vi "lorentzian transformations--test.vi"() -> ()   [LabVIEW 2020]
uses:
  lorentzian.ctl
  circle corners.ctl
  cursor action.ctl
  four-corner circle transformation.ctl
  Q -- check range -- i -- real.vi
  draw a line.vi
  draw a circle.vi
  Q - not nan -- real.vi
  generate linear region.vi
panel:
  in  "lorentzian hist":T1={"A (VHz)"=1.0, "f (Hz)"=900.0, "G (Hz)"=10.0, "phi(rad)"=0.0, "Q"=0.006429595340103388, "Norm  Ampl"=nan, "bg (V)"=0.0+0.0i, "4corners"={"z (-pi/2)"=0.1-0.1i, "z(inf)"=0.0+0.0i, "z (pi/2)"=-0.1-0.1i, "z center"=0.0-0.1i, "z(0)"=0.0-0.2i, "radius"=0.1}} {"bg (V)" format="%#9_9f"; "Q" format="%#9_9f"; "phi(rad)" format="%#9_9f"; "G (Hz)" format="%#9_9f"; "f (Hz)" format="%#9_9f"}
  in  "Tab Control":enum32{"Page 1", "Page 2"}(tab)
  in  "phase":dbl(slide) scale=-1.57..1.57
  out "Plot: complex plane":cluster{dbl[], dbl[]}[](graph)=[{[0.1, 0.09991228300988585, 0.09964928592495044, 0.0992114701314478, 0.0985996037070505, 0.09781476007338057, 0.09685831611286312, 0.09573194975320673, 0.0944376370237481, 0.09297764858882515, 0.0913545457642601, 0.0895711760239413, 0.08763066800438636, 0.08553642601605067, 0.08329212407100996, 0.08090169943749474, 0.07836934573258399, 0.07569950556517566, 0.07289686274214116, 0.06996633405133655, 0.06691306063588583, 0.06374239897486898, 0.06045991148623749, 0.05707135676844318, 0.05358267949789968, 0.05000000000000001, 0.04632960351198618, 0.04257792915650729, 0.038751558645210314, 0.03485720473218153, 0.03090169943749475, 0.02689198206152659, 0.02283508701106559, 0.018738131458572473, 0.014608302856241187, 0.010452846326765368, 0.006279051952931353, 0.002094241988335705, -0.0020942419883356704, -0.006279051952931318, -0.010452846326765334, -0.014608302856241132, -0.01873813145857244, -0.02283508701106556, -0.02689198206152656, -0.030901699437494715, -0.0348572047321815, -0.03875155864521028, -0.04257792915650724, -0.04632960351198615, -0.04999999999999998, -0.05358267949789965, -0.05707135676844316, -0.060459911486237486, -0.06374239897486894, -0.0669130606358858, -0.06996633405133652, -0.07289686274214113, -0.07569950556517563, -0.07836934573258397, -0.08090169943749474, -0.08329212407100993, -0.08553642601605065, -0.08763066800438635, -0.08957117602394128, -0.09135454576426008, -0.09297764858882514, -0.0944376370237481, -0.09573194975320672, -0.09685831611286311, -0.09781476007338057, -0.0985996037070505, -0.09921147013144778, -0.09964928592495044, -0.09991228300988585, -0.1, -0.09991228300988585, -0.09964928592495044, -0.0992114701314478, -0.09859960370705051, -0.09781476007338058, -0.09685831611286312, -0.09573194975320674, -0.09443763702374813, -0.09297764858882517, -0.09135454576426011, -0.08957117602394131, -0.08763066800438638, -0.08553642601605069, -0.08329212407100998, -0.08090169943749478, -0.07836934573258401, -0.07569950556517568, -0.07289686274214119, -0.06996633405133657, -0.06691306063588585, -0.06374239897486902, -0.06045991148623754, -0.05707135676844322, -0.05358267949789971, -0.050000000000000044, -0.046329603511986214, -0.0425779291565073, -0.03875155864521033, -0.03485720473218155, -0.03090169943749476, -0.026891982061526584, -0.022835087011065666, -0.01873813145857255, -0.014608302856241245, -0.010452846326765424, -0.006279051952931409, -0.002094241988335762, 0.002094241988335636, 0.006279051952931284, 0.010452846326765299, 0.01460830285624112, 0.018738131458572428, 0.022835087011065545, 0.026891982061526546, 0.030901699437494726, 0.03485720473218143, 0.03875155864521021, 0.04257792915650718, 0.0463296035119861, 0.04999999999999993, 0.053582679497899605, 0.05707135676844312, 0.06045991148623744, 0.06374239897486893, 0.06691306063588578, 0.06996633405133651, 0.07289686274214113, 0.07569950556517563, 0.07836934573258397, 0.08090169943749473, 0.0832921240710099, 0.08553642601605062, 0.08763066800438632, 0.08957117602394125, 0.09135454576426007, 0.09297764858882512, 0.09443763702374809, 0.09573194975320672, 0.09685831611286311, 0.09781476007338055, 0.0985996037070505, 0.09921147013144778, 0.09964928592495044, 0.09991228300988583], [-0.1, -0.09581243462708004, -0.09163221566676846, -0.08746667664356958, -0.08332312532838979, -0.07920883091822407, -0.07513101128351453, -0.07109682030555285, -0.0671133353261417, -0.06318754473153221, -0.05932633569241998, -0.05553648208150726, -0.05182463258982848, -0.04819729906268699, -0.0446608450756656, -0.04122147477075269, -0.037885221972168974, -0.034657939600989465, -0.03154528940713114, -0.02855273203671968, -0.02568551745226058, -0.022948675722421083, -0.020347008197580382, -0.017885079086629604, -0.015567207449798504, -0.01339745962155614, -0.011379642076878527, -0.009517294753398062, -0.007813684841149957, -0.006271801050810849, -0.00489434837048465, -0.0036837433202341896, -0.002642109712683971, -0.001771274927131139, -0.0010727667037011696, -0.0005478104631726627, -0.00019732715717284133, -2.1931652515447264e-05, -2.1931652515447264e-05, -0.00019732715717284133, -0.0005478104631726627, -0.0010727667037011696, -0.0017712749271311251, -0.002642109712683971, -0.0036837433202341757, -0.004894348370484636, -0.006271801050810835, -0.007813684841149943, -0.009517294753398034, -0.011379642076878513, -0.013397459621556126, -0.01556720744979849, -0.01788507908662959, -0.02034700819758037, -0.022948675722421055, -0.025685517452260553, -0.02855273203671964, -0.03154528940713111, -0.03465793960098944, -0.03788522197216895, -0.041221474770752685, -0.044660845075665555, -0.048197299062686945, -0.051824632589828445, -0.05553648208150723, -0.05932633569241996, -0.06318754473153218, -0.06711333532614167, -0.0710968203055528, -0.07513101128351449, -0.07920883091822403, -0.08332312532838974, -0.08746667664356955, -0.09163221566676844, -0.09581243462708003, -0.09999999999999995, -0.10418756537291991, -0.1083677843332315, -0.11253332335643039, -0.1166768746716102, -0.12079116908177591, -0.12486898871648547, -0.12890317969444712, -0.1328866646738583, -0.13681245526846775, -0.14067366430758, -0.1444635179184927, -0.1481753674101715, -0.15180270093731302, -0.15533915492433437, -0.15877852522924726, -0.162114778027831, -0.1653420603990105, -0.16845471059286884, -0.1714472679632803, -0.1743144825477394, -0.1770513242775789, -0.17965299180241961, -0.1821149209133704, -0.1844327925502015, -0.18660254037844387, -0.18862035792312146, -0.19048270524660194, -0.19218631515885004, -0.19372819894918913, -0.19510565162951538, -0.19631625667976582, -0.197357890287316, -0.19822872507286887, -0.19892723329629883, -0.19945218953682733, -0.19980267284282716, -0.19997806834748455, -0.19997806834748455, -0.19980267284282716, -0.19945218953682736, -0.19892723329629886, -0.19822872507286887, -0.19735789028731604, -0.19631625667976582, -0.19510565162951538, -0.1937281989491892, -0.1921863151588501, -0.190482705246602, -0.18862035792312154, -0.18660254037844393, -0.18443279255020156, -0.18211492091337045, -0.17965299180241967, -0.17705132427757897, -0.17431448254773946, -0.17144726796328036, -0.1684547105928689, -0.16534206039901056, -0.16211477802783106, -0.15877852522924735, -0.1553391549243345, -0.15180270093731313, -0.14817536741017162, -0.14446351791849282, -0.1406736643075801, -0.13681245526846786, -0.1328866646738584, -0.12890317969444723, -0.12486898871648554, -0.12079116908177599, -0.11667687467161028, -0.11253332335643047, -0.10836778433323159, -0.10418756537292]}, {[0.0, 0.0, 0.0, 0.0, 0.0, 0.0, 0.0, 0.0, 0.0, 0.0, 0.0, 0.0, 0.0, 0.0, 0.0, 0.0, 0.0, 0.0, 0.0, 0.0], [0.0, -0.01, -0.02, -0.03, -0.04, -0.05, -0.06, -0.07, -0.08, -0.09, -0.1, -0.11, -0.12, -0.13, -0.14, -0.15, -0.16, -0.17, -0.18, -0.19]}, {[0.1, 0.09000000000000001, 0.08, 0.07, 0.060000000000000005, 0.05, 0.04000000000000001, 0.03, 0.020000000000000004, 0.010000000000000009, 0.0, -0.009999999999999995, -0.01999999999999999, -0.03, -0.04000000000000001, -0.04999999999999999, -0.06, -0.07, -0.07999999999999999, -0.09], [-0.1, -0.1, -0.1, -0.1, -0.1, -0.1, -0.1, -0.1, -0.1, -0.1, -0.1, -0.1, -0.1, -0.1, -0.1, -0.1, -0.1, -0.1, -0.1, -0.1]}, {[0.2, 0.18000000000000002, 0.16, 0.14, 0.12000000000000001, 0.1, 0.08000000000000002, 0.06, 0.04000000000000001, 0.020000000000000018, 0.0, -0.01999999999999999, -0.03999999999999998, -0.06, -0.08000000000000002, -0.09999999999999998, -0.12, -0.14, -0.15999999999999998, -0.18], [-1.2246063538223773e-17, -1.2246063538223773e-17, -1.2246063538223773e-17, -1.2246063538223773e-17, -1.2246063538223773e-17, -1.2246063538223773e-17, -1.2246063538223773e-17, -1.2246063538223773e-17, -1.2246063538223773e-17, -1.2246063538223773e-17, -1.2246063538223773e-17, -1.2246063538223773e-17, -1.2246063538223773e-17, -1.2246063538223773e-17, -1.2246063538223773e-17, -1.2246063538223773e-17, -1.2246063538223773e-17, -1.2246063538223773e-17, -1.2246063538223773e-17, -1.2246063538223773e-17]}]
  in  "lorentzian":T1={"A (VHz)"=1.0, "f (Hz)"=900.0, "G (Hz)"=10.0, "phi(rad)"=0.0, "Q"=0.006429595340103388, "Norm  Ampl"=nan, "bg (V)"=0.0+0.0i, "4corners"={"z (-pi/2)"=0.1-0.1i, "z(inf)"=0.0+0.0i, "z (pi/2)"=-0.1-0.1i, "z center"=0.0-0.1i, "z(0)"=0.0-0.2i, "radius"=0.1}} {"bg (V)" format="%#9_9f"; "Q" format="%#9_9f"; "phi(rad)" format="%#9_9f"; "G (Hz)" format="%#9_9f"; "f (Hz)" format="%#9_9f"}
  in  "exit":bool
  in  "omega":dbl(slide)=911.4832535885167 scale=500.0..1500.0
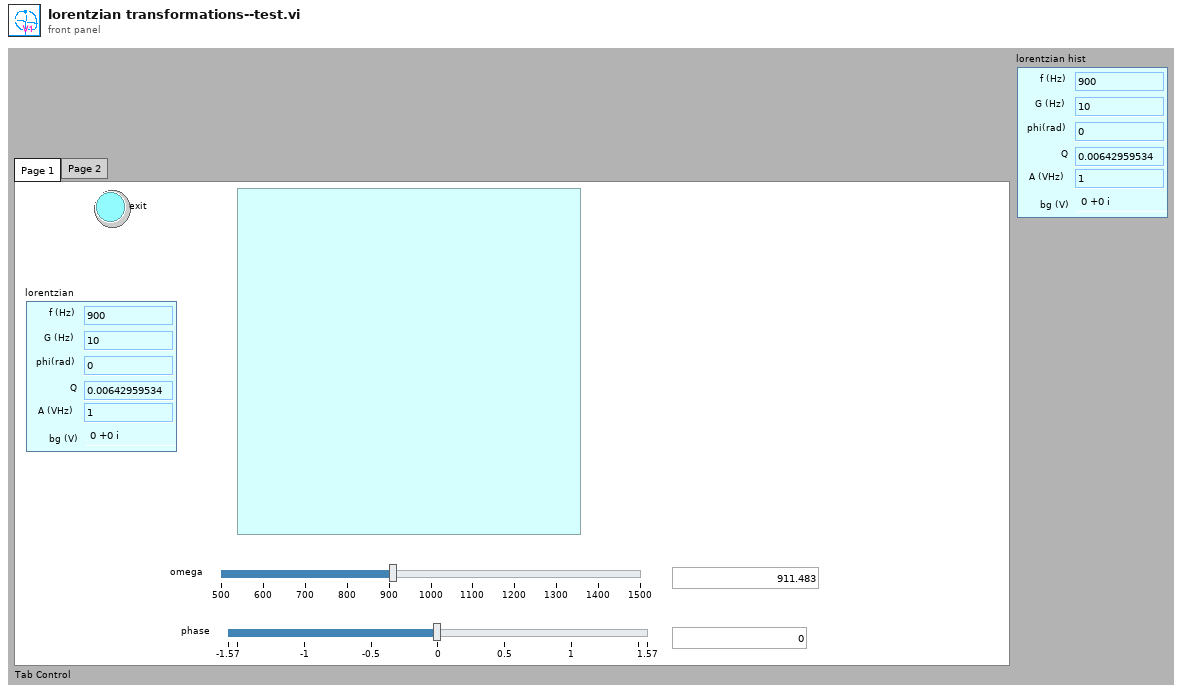
[diagram p1: front panel]
types:
  T1 = typedef "lorentzian.ctl" = cluster{"A (VHz)":dbl, "f (Hz)":dbl, "G (Hz)":dbl, "phi(rad)":dbl, "Q":dbl, "Norm  Ampl":dbl, "bg (V)":cdb, "4corners":T2}
  T2 = typedef "circle corners.ctl" = cluster{"z (-pi/2)":cdb, "z(inf)":cdb, "z (pi/2)":cdb, "z center":cdb, "z(0)":cdb, "radius":dbl}
  T3 = typedef "four-corner circle transformation.ctl" = enum16{"z(c) z(inf)", "z(c) z(zero)", "fix phase", "calculate lorentzian", "z(0) z(+-pi/2)", "shift to zcenter", "to  canonical", "get canonical phase", "get4corners", "update lorentzian -- from z0", "fake gamma normal", "fake gamma heat", "calculate complex slope", "get f0 given f and phi"}
  T4 = typedef "cursor action.ctl" = enum16{"range", "read", "write", "check", "zoom out", "smart zoom out", "zoom to aspect ratio 1", "zoom to win", "zoom out 20%", "zoom in 20%", "-empty", "smart zoom out&aspect", "move range left 20%", "move range right 20%", "move range up 20%", "move range down 20%", "zoom to X win", "zoom to Y win", "zoom out X", "zoom out Y", "zoom in X", "zoom in Y", "check plot scale"}
  T5 = typedef "eventvkey.ctl" = enum16{"ASCII", "Enter", "Return", "Shift", "Ctrl", "Alt", "Cmd", "Opt", "Caps", "NumLock", "Clear", "Break", "Up", "Down", "Left", "Right", "Insert", "Delete", "Home", "End", "PageUp", "PageDown", "Escape", "Help", "Pause", "ScrollLock", "F1", "F2", "F3", "F4", "F5", "F6", "F7", "F8", "F9", "F10", "F11", "F12", "F13", "F14", "F15", "F16", "F17", "F18", "F19", "F20", "F21", "F22", "F23", "F24", "Play", "VolumeUp", "VolumeDown", "Mute", "Two Byte Char"}
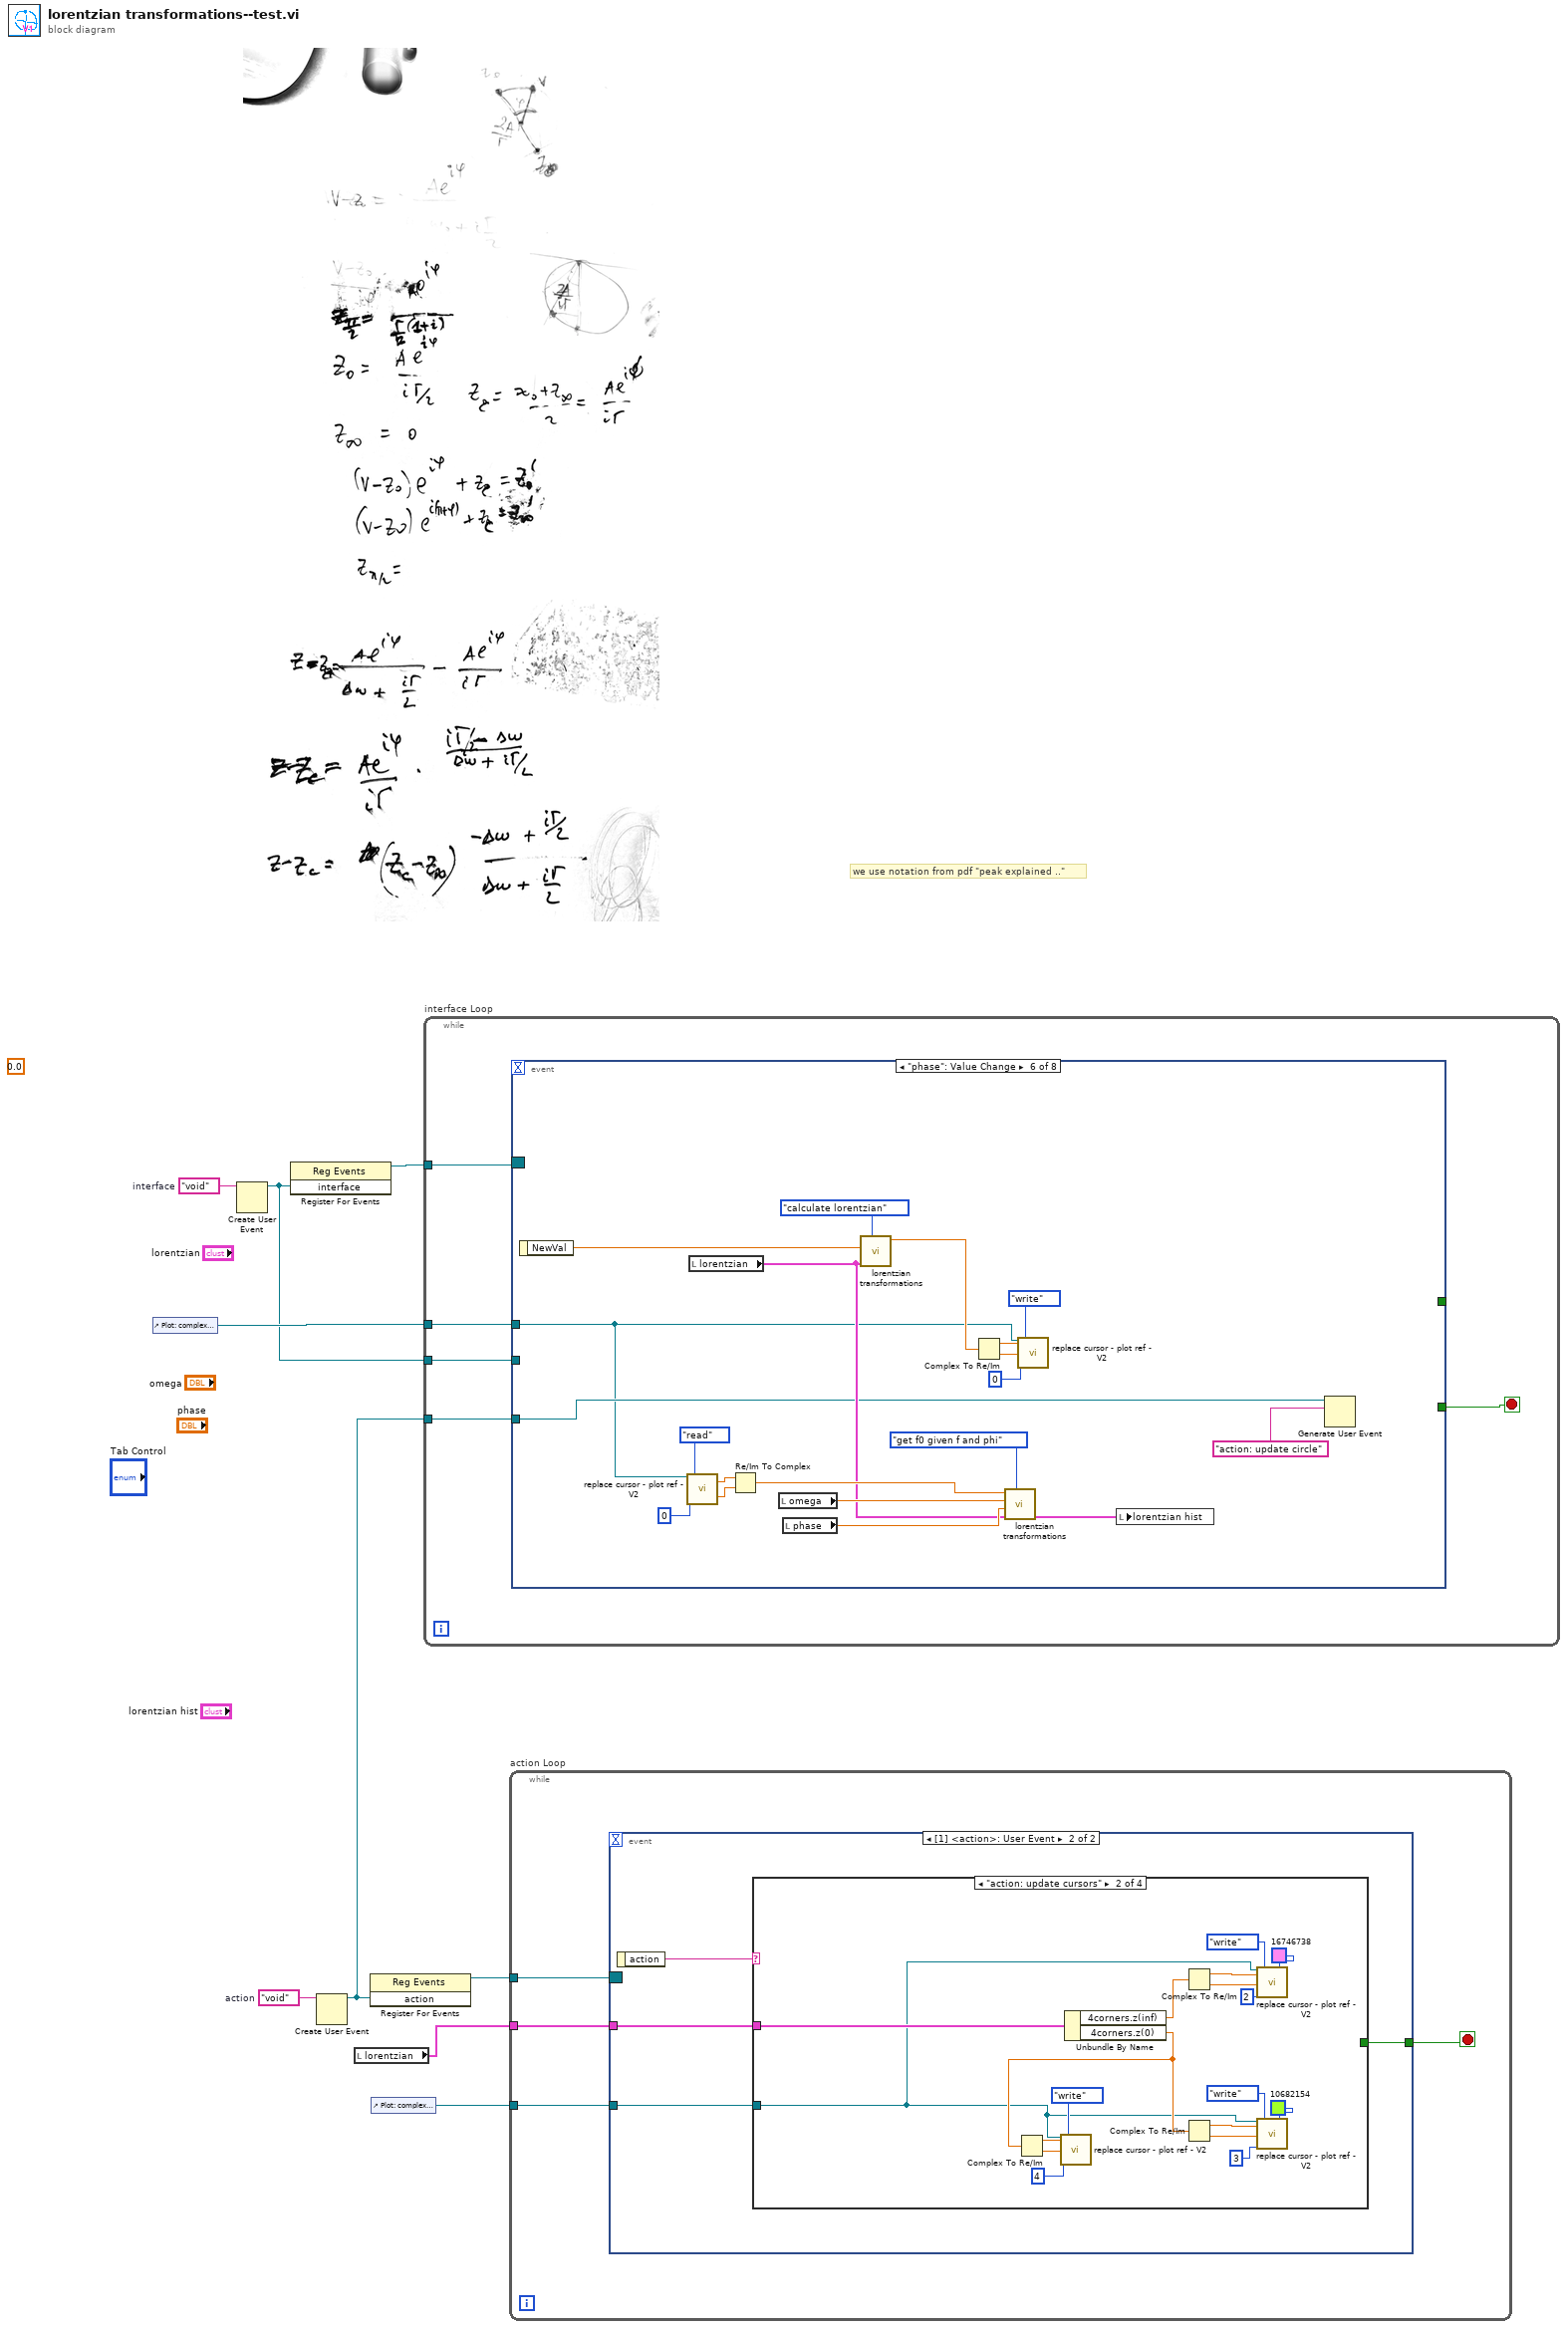
[diagram p0: block diagram]
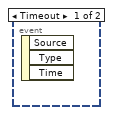
[diagram p2: hidden frame]
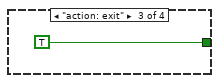
[diagram p4: hidden frame]
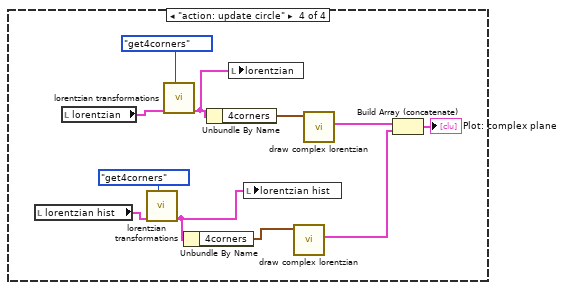
[diagram p5: hidden frame]
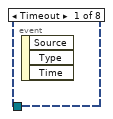
[diagram p6: hidden frame]
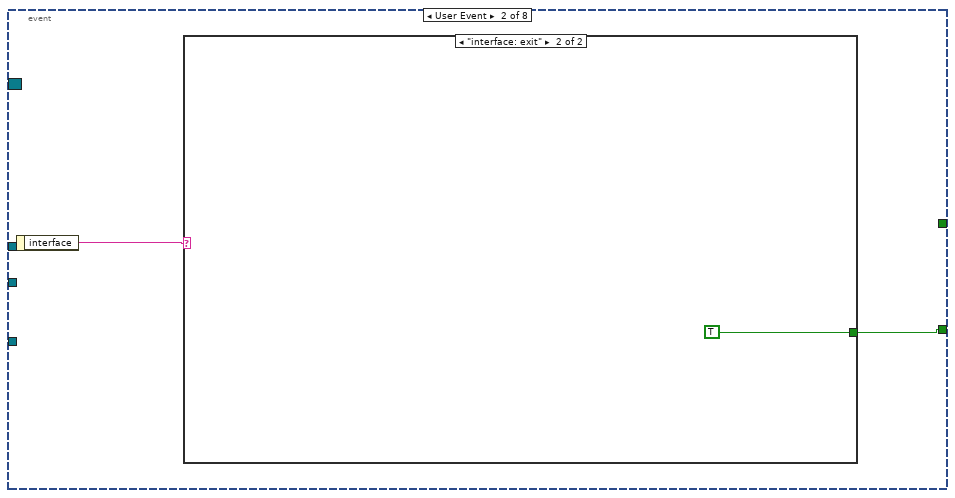
[diagram p7: hidden frame]
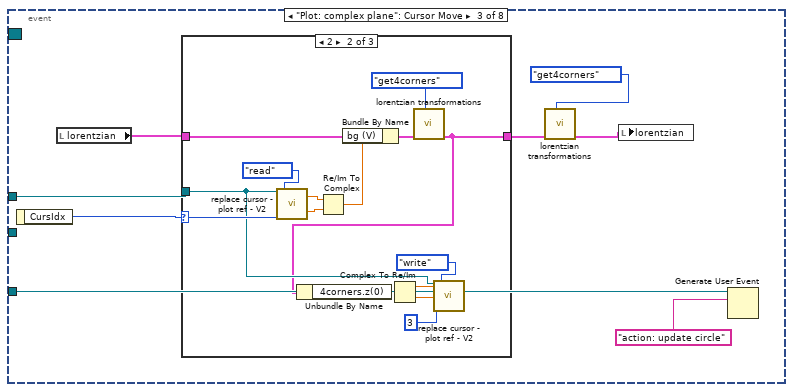
[diagram p9: hidden frame]
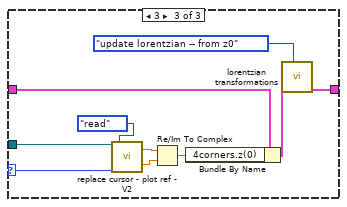
[diagram p11: hidden frame]
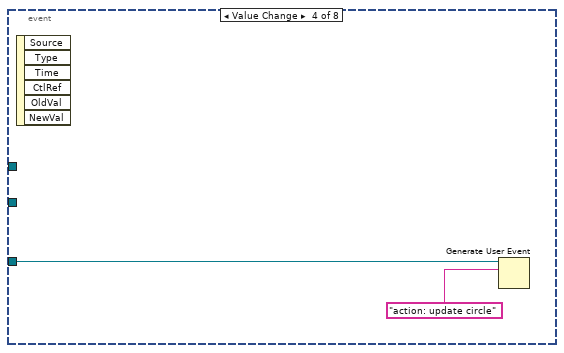
[diagram p12: hidden frame]
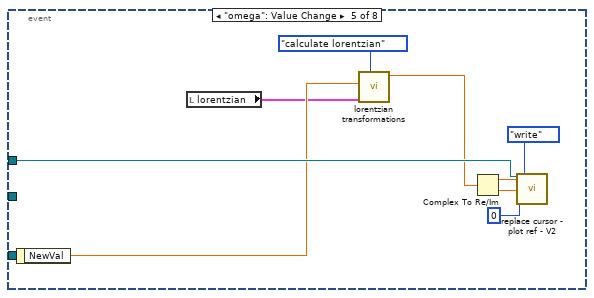
[diagram p13: hidden frame]
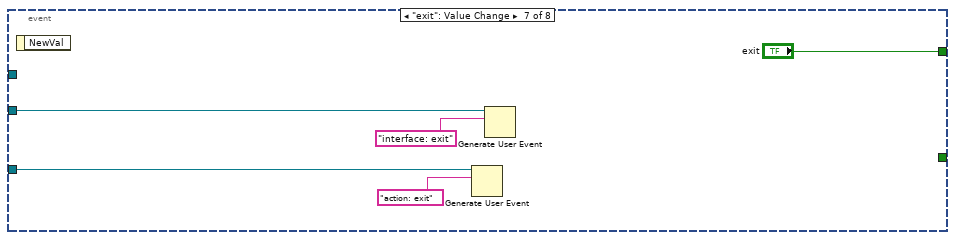
[diagram p14: hidden frame]
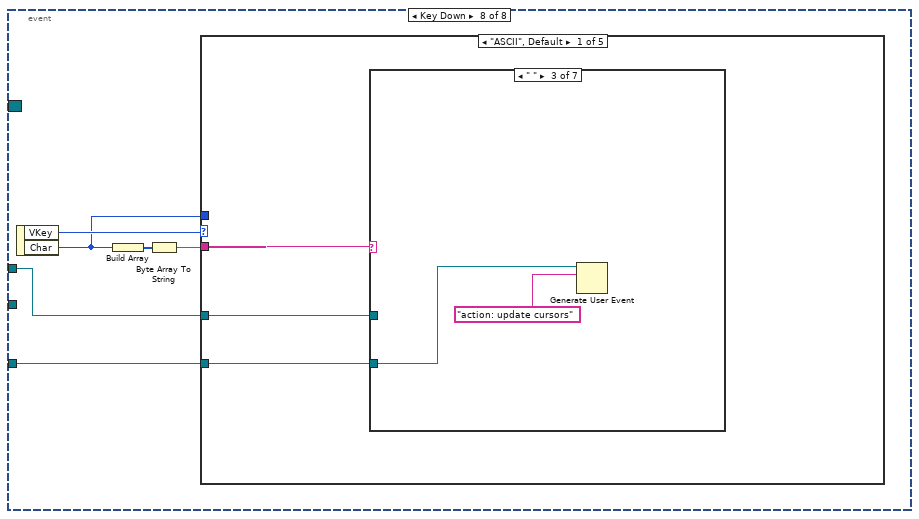
[diagram p15: hidden frame]
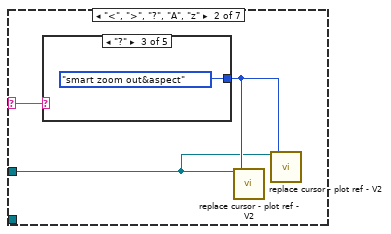
[diagram p17: hidden frame]
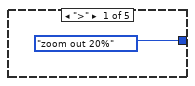
[diagram p18: hidden frame]
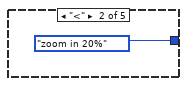
[diagram p19: hidden frame]
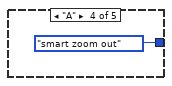
[diagram p20: hidden frame]
diagram:
  w5 = "void"  # interface
  w9 = "void"  # action
  (unwired) 0.0 ("zi phase temporary")
  # "we use notation from pdf \"peak explained ..\""
  n1 = control-ref of="Plot: complex plane"() -> (w2:refnum<vi>)
  n2 = Create User Event(user event datatype=w5) -> (user event=w1:refnum<user-event>)  [unwired: 1 in, 1 out]
  n3 = register-events(w1) -> (reference out=w4:refnum<event-registration>)  [unwired: 2 in, 1 out]
  n4 = Create User Event(user event datatype=w9) -> (user event=w3:refnum<user-event>)  [unwired: 1 in, 1 out]
  n5 = local read "lorentzian"() -> (w6:T1)
  n6 = register-events(w3) -> (reference out=w8:refnum<event-registration>)  [unwired: 2 in, 1 out]
  n7 = control-ref of="Plot: complex plane"() -> (w7:refnum<vi>)
  n8 = while "interface Loop" {
    tunnel: w4 -> [w14]
    tunnel: w3 -> [w13]
    tunnel: w2 -> [w12]
    tunnel: w1 -> [w10]
    stop <- w11 stop-if-true
    n9 = event shown="[5] \"phase\": Value Change" {
      selector: w14 -> [_ _ _ _ _ _ _ _]
      dyn-events: _ -> [_ _ _ _ _ _ _ _]
      timeout: _ -> [_ _ _ _ _ _ _ _]
      tunnel: [_ _ _ _ _ _ "exit" _] -> _
      tunnel: w13 -> [_ _ w18 w52 _ w64 w85 w88]
      tunnel: w12 -> [_ _ w22 _ w57 w63 _ w89]
      tunnel: [_ w15 _ _ _ _ _ _] -> w11
      tunnel: w10 -> [_ _ _ _ _ _ w83 _]
      event Timeout {
        n10 = event-data() -> ()  [unwired: 1 in, 3 out]
      }
      event User Event {
        n11 = event-data() -> ("interface"=w16:string)  [unwired: 1 in]
        n12 = case shown="\"interface: exit\"" w16 {
          tunnel: [_ TRUE] -> w15
          frame "False", Default {
          }
          frame "interface: exit" {
          }
        }
      }
      event "Plot: complex plane": Cursor Move {
        n13 = event-data() -> ("CursIdx"=w21:i32)  [unwired: 1 in]
        n14 = local read "lorentzian"() -> (w23:T1)
        n15 = case shown="2" w21 {
          selector: w21 -> [_ w37 w47]
          tunnel: w22 -> [_ w31 w46]
          tunnel: w23 -> [w26 w27 w45]
          tunnel: [w26 w28 w42] -> w25
          frame 0, Default {
          }
          frame 2 {
            n16 = call "replace cursor - plot ref - V2.vi"("Plot ref in"=w31, "cursor index"=w37, "cursor action"=cursor_action."read") -> ("read X"=w39:dbl, "read Y"=w40:dbl)  [unwired: 13 in, 2 out]
            n17 = Re/Im To Complex(1:w40, 2:w39) -> (0:w38:cdb)
            n18 = Bundle By Name(cluster=w27, "bg (V)"=w38) -> (w36:T1)
            n19 = call "lorentzian transformations.vi"("4 corner circle transformation"=four-corner_circle_transformation."get4corners", "lorentzian in"=w36) -> ("lorentzian out"=w28:T1)  [unwired: 6 in, 3 out]
            n20 = Unbundle By Name(w28) -> ("4corners.z(0)"=w34:cdb)
            n21 = Complex To Re/Im(x + iy=w34) -> (x=w33:dbl, y=w32:dbl)
            n22 = call "replace cursor - plot ref - V2.vi"("Plot ref in"=w31, "new X"=w33, "new  Y"=w32, "cursor index"=3, "cursor action"=cursor_action."write") -> ()  [unwired: 11 in, 4 out]
          }
          frame 3 {
            n23 = call "replace cursor - plot ref - V2.vi"("Plot ref in"=w46, "cursor index"=w47, "cursor action"=cursor_action."read") -> ("read X"=w49:dbl, "read Y"=w50:dbl)  [unwired: 13 in, 2 out]
            n24 = Re/Im To Complex(1:w50, 2:w49) -> (0:w48:cdb)
            n25 = Bundle By Name(cluster=w45, "4corners.z(0)"=w48) -> (w44:T1)
            n26 = call "lorentzian transformations.vi"("4 corner circle transformation"=four-corner_circle_transformation."update lorentzian -- from z0", "lorentzian in"=w44) -> ("lorentzian out"=w42:T1)  [unwired: 6 in, 3 out]
          }
        }
        n27 = call "lorentzian transformations.vi"("4 corner circle transformation"=four-corner_circle_transformation."get4corners", "lorentzian in"=w25) -> ("lorentzian out"=w20:T1)  [unwired: 6 in, 3 out]
        n28 = local write "lorentzian"(w20) -> ()
        n29 = Generate User Event(user event=w18, event data cluster="action: update circle" ("event data")) -> ()  [unwired: 2 in, 2 out]
      }
      event Value Change {
        n30 = event-data() -> ()  [unwired: 1 in, 6 out]
        n31 = Generate User Event(user event=w52, event data cluster="action: update circle" ("event data")) -> ()  [unwired: 2 in, 2 out]
      }
      event "omega": Value Change {
        n32 = event-data() -> ("NewVal"=w55:dbl)  [unwired: 1 in]
        n33 = local read "lorentzian"() -> (w54:T1)
        n34 = call "lorentzian transformations.vi"("4 corner circle transformation"=four-corner_circle_transformation."calculate lorentzian", "lorentzian in"=w54, "freq in"=w55) -> ("voltage out"=w56:cdb)  [unwired: 5 in, 3 out]
        n35 = Complex To Re/Im(x + iy=w56) -> (x=w61:dbl, y=w60:dbl)
        n36 = call "replace cursor - plot ref - V2.vi"("Plot ref in"=w57, "new X"=w61, "new  Y"=w60, "cursor index"=0, "cursor action"=cursor_action."write") -> ()  [unwired: 11 in, 4 out]
      }
      event "phase": Value Change {
        n37 = event-data() -> ("NewVal"=w76:dbl)  [unwired: 1 in]
        n38 = call "replace cursor - plot ref - V2.vi"("Plot ref in"=w63, "cursor index"=0, "cursor action"=cursor_action."read") -> ("read X"=w71:dbl, "read Y"=w72:dbl)  [unwired: 13 in, 2 out]
        n39 = local read "lorentzian"() -> (w68:T1)
        n40 = Re/Im To Complex(1:w72, 2:w71) -> (0:w70:cdb)
        n41 = local read "omega"() -> (w75:dbl)
        n42 = local read "phase"() -> (w69:dbl)
        n43 = call "lorentzian transformations.vi"("4 corner circle transformation"=four-corner_circle_transformation."calculate lorentzian", "lorentzian in"=w68, "freq in"=w76) -> ("voltage out"=w77:cdb)  [unwired: 5 in, 3 out]
        n44 = Complex To Re/Im(x + iy=w77) -> (x=w81:dbl, y=w80:dbl)
        n45 = call "lorentzian transformations.vi"("4 corner circle transformation"=four-corner_circle_transformation."get f0 given f and phi", "lorentzian in"=w68, "phase in (rad)"=w69, "freq in"=w75, "voltage in"=w70) -> ("lorentzian out"=w67:T1)  [unwired: 3 in, 3 out]
        n46 = call "replace cursor - plot ref - V2.vi"("Plot ref in"=w63, "new X"=w81, "new  Y"=w80, "cursor index"=0, "cursor action"=cursor_action."write") -> ()  [unwired: 11 in, 4 out]
        n47 = local write "lorentzian hist"(w67) -> ()
        n48 = Generate User Event(user event=w64, event data cluster="action: update circle" ("event data")) -> ()  [unwired: 2 in, 2 out]
      }
      event "exit": Value Change {
        n49 = event-data() -> ()  [unwired: 1 in, 1 out]
        n50 = Generate User Event(user event=w85, event data cluster="action: exit" ("event data")) -> ()  [unwired: 2 in, 2 out]
        n51 = Generate User Event(user event=w83, event data cluster="interface: exit" ("event data")) -> ()  [unwired: 2 in, 2 out]
      }
      event Key Down {
        n52 = event-data() -> ("VKey"=w91:T5, "Char"=w90:i16)  [unwired: 1 in]
        n53 = Build Array(w90) -> (w93:i16[])
        n54 = Byte Array To String(unsigned byte array=w93) -> (string=w92:string)
        n55 = case shown="\"ASCII\", Default" w91 {
          selector: w91 -> [_ _ _ _ w109]
          tunnel: w90 -> [_ _ _ _ _]
          tunnel: w92 -> [w96 _ _ _ _]
          tunnel: w89 -> [w95 _ _ _ w107]
          tunnel: w88 -> [w94 _ _ _ _]
          frame "ASCII", Default {
            n56 = case shown="\" \"" w96 {
              selector: w96 -> [_ w98 _ _ _ _ _]
              tunnel: w95 -> [_ w97 _ _ _ _ _]
              tunnel: w94 -> [_ _ w105 _ _ _ _]
              frame "0", Default {
              }
              frame "<", ">", "?", "A", "z" {
                n57 = case shown="\"?\"" w98 {
                  tunnel: [cursor_action."zoom out 20%" ("cursor action") cursor_action."zoom in 20%" ("cursor action") cursor_action."smart zoom out&aspect" ("cursor action") cursor_action."smart zoom out" ("cursor action") cursor_action."zoom to aspect ratio 1" ("cursor action")] -> w99
                  frame ">" {
                  }
                  frame "<" {
                  }
                  frame "?" {
                  }
                  frame "A" {
                  }
                  frame "z", Default {
                  }
                }
                n58 = call "replace cursor - plot ref - V2.vi"("Plot ref in"=w97, "cursor action"=w99) -> ()  [unwired: 14 in, 4 out]
                n59 = call "replace cursor - plot ref - V2.vi"("Plot ref in"=w97, "cursor action"=w99) -> ()  [unwired: 14 in, 4 out]
              }
              frame " " {
                n60 = Generate User Event(user event=w105, event data cluster="action: update cursors" ("event data")) -> ()  [unwired: 2 in, 2 out]
              }
              frame "'", ";", "[", "]", "{", "}" {
              }
              frame "@" {
              }
              frame "#" {
              }
              frame "q" {
              }
            }
          }
          frame "Escape" {
          }
          frame "PageUp" {
          }
          frame "PageDown" {
          }
          frame "Up".."Right" {
            n61 = case shown="\"Down\"" w109 {
              tunnel: [cursor_action."move range right 20%" ("cursor action") cursor_action."move range left 20%" ("cursor action") cursor_action."move range up 20%" ("cursor action") cursor_action."move range down 20%" ("cursor action")] -> w108
              frame "Right", Default {
              }
              frame "Left" {
              }
              frame "Up" {
              }
              frame "Down" {
              }
            }
            n62 = call "replace cursor - plot ref - V2.vi"("Plot ref in"=w107, "cursor action"=w108) -> ()  [unwired: 14 in, 4 out]
            n63 = call "replace cursor - plot ref - V2.vi"("Plot ref in"=w107, "cursor action"=w108) -> ()  [unwired: 14 in, 4 out]
          }
        }
      }
    }
  }
  n64 = while "action Loop" {
    tunnel: w8 -> [w117]
    tunnel: w7 -> [w116]
    tunnel: w6 -> [w115]
    stop <- w114 stop-if-true
    n65 = event shown="[1] <action>: User Event" {
      selector: w117 -> [_ _]
      dyn-events: _ -> [_ _]
      timeout: _ -> [_ _]
      tunnel: w116 -> [_ w120]
      tunnel: w115 -> [_ w119]
      tunnel: [_ w118] -> w114
      event Timeout {
        n66 = event-data() -> ()  [unwired: 1 in, 3 out]
      }
      event User Event {
        n67 = event-data() -> ("action"=w121:string)  [unwired: 1 in]
        n68 = case shown="\"action: update cursors\"" w121 {
          tunnel: w120 -> [_ w122 _ _]
          tunnel: w119 -> [_ w128 _ _]
          tunnel: [_ _ TRUE _] -> w118
          frame "False", Default {
          }
          frame "action: update cursors" {
            n69 = Unbundle By Name(w128) -> ("4corners.z(inf)"=w137:cdb, "4corners.z(0)"=w123:cdb)
            n70 = Complex To Re/Im(x + iy=w123) -> (x=w127:dbl, y=w126:dbl)
            n71 = call "replace cursor - plot ref - V2.vi"("Plot ref in"=w122, "new X"=w127, "new  Y"=w126, "cursor index"=4, "cursor action"=cursor_action."write") -> ()  [unwired: 11 in, 4 out]
            n72 = Complex To Re/Im(x + iy=w137) -> (x=w135:dbl, y=w136:dbl)
            n73 = Complex To Re/Im(x + iy=w123) -> (x=w138:dbl, y=w139:dbl)
            n74 = call "replace cursor - plot ref - V2.vi"("Plot ref in"=w122, "new X"=w135, "new  Y"=w136, "cursor index"=2, "cursor action"=cursor_action."write", "Color Box"=u32 16746738) -> ()  [unwired: 10 in, 4 out]
            n75 = call "replace cursor - plot ref - V2.vi"("Plot ref in"=w122, "new X"=w138, "new  Y"=w139, "cursor index"=3, "cursor action"=cursor_action."write", "Color Box"=u32 10682154) -> ()  [unwired: 10 in, 4 out]
          }
          frame "action: exit" {
          }
          frame "action: update circle" {
            n76 = local read "lorentzian hist"() -> (w146:T1)
            n77 = local read "lorentzian"() -> (w150:T1)
            n78 = call "lorentzian transformations.vi"("4 corner circle transformation"=four-corner_circle_transformation."get4corners", "lorentzian in"=w146) -> ("lorentzian out"=w145:T1)  [unwired: 6 in, 3 out]
            n79 = call "lorentzian transformations.vi"("4 corner circle transformation"=four-corner_circle_transformation."get4corners", "lorentzian in"=w150) -> ("lorentzian out"=w149:T1)  [unwired: 6 in, 3 out]
            n80 = Unbundle By Name(w145) -> ("4corners"=w144:T2)
            n81 = Unbundle By Name(w149) -> ("4corners"=w151:T2)
            n82 = local write "lorentzian"(w149) -> ()
            n83 = local write "lorentzian hist"(w145) -> ()
            n84 = call "draw complex lorentzian.vi"("4 corners"=w144) -> ("fancy circles"=w142:cluster{dbl[], dbl[]}[])  [unwired: 10 in]
            n85 = call "draw complex lorentzian.vi"("4 corners"=w151) -> ("fancy circles"=w143:cluster{dbl[], dbl[]}[])  [unwired: 10 in]
            n86 = Build Array (concatenate)(w143, w142) -> (→"Plot: complex plane":cluster{dbl[], dbl[]}[])
          }
        }
      }
    }
  }
